vi "do_Weight_Weighing_Machine.vi"(8 "error in (no error)":errorcluster, 11 "Waage_Config":T1={"Enable Termination\nChar (T)"=TRUE, "termination char\n(0xA = '\\n' = LF) "=10, "timeout (10sec)"=3000, "baud rate (9600)"=9600, "data bits (8)"=8, "parity (0:none)"=enum."None", "stop bits (10: 1 bit)"=10, "flow control (0:none)"=0, "Serial Port"=""} {"flow control (0:none)" items=["None", "XON/XOFF", "RTS/CTS", "XON/XOFF & RTS/CTS", "DTR/DSR", "XON/XOFF & DTR/DSR"]; "stop bits (10: 1 bit)" items=["1.0"=10, "1.5"=15, "2.0"=20]}) -> (0 "error out":errorcluster={"status"=TRUE, "code"=-1073807339, "source"="VISA Read in do_Weight_Weighing_Machine.vi"}, 3 "weight(g)":i32)   [LabVIEW 2012]
uses:
  <vilib>/Instr/_visa.llb/VISA Configure Serial Port (Instr).vi
panel:
  out "return count 2":u32=9
  out "return count":u32
  out "read buffer":string
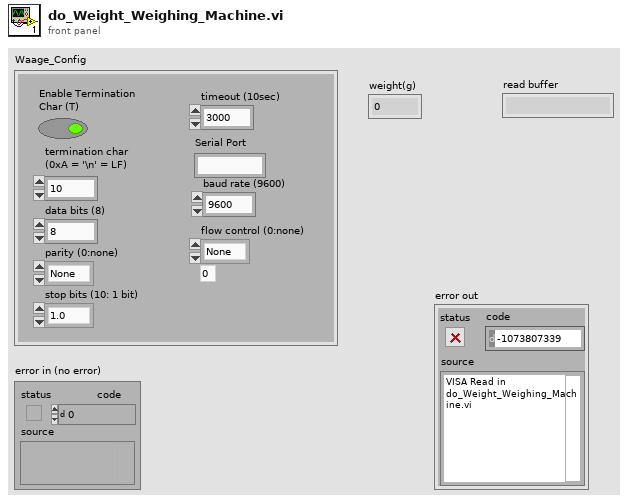
[diagram p1: front panel]
types:
  T1 = cluster{"Enable Termination\nChar (T)":bool, "termination char\n(0xA = '\\n' = LF) ":u8, "timeout (10sec)":u32, "baud rate (9600)":u32, "data bits (8)":u16, "parity (0:none)":enum16{"None", "Odd", "Even", "Mark", "Space"}, "stop bits (10: 1 bit)":u16, "flow control (0:none)":u16, "Serial Port":string}
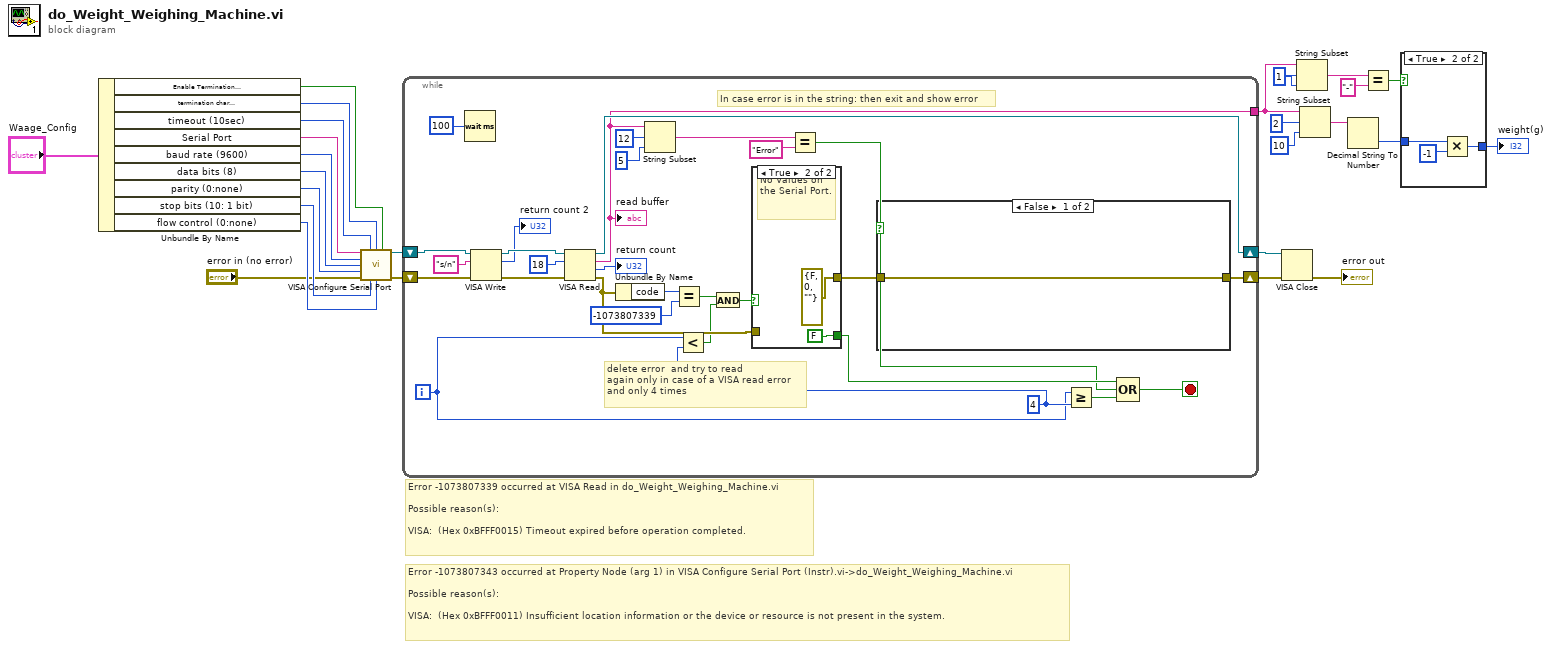
[diagram p0: block diagram]
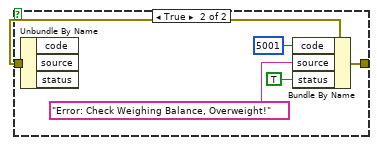
[diagram p3: hidden frame]
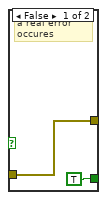
[diagram p4: hidden frame]
diagram:
  w11 = 1 ("offset (0)")
  # "Error -1073807343 occurred at Property Node (arg 1) in VISA Configure Serial Port (Instr).vi->do_Weight_Weighing_Machine.vi\n\nPossible reason(s):\n\nVISA:  (Hex 0xBFFF0011) Insufficient location information or the device or resource is not present in the system."
  # "Error -1073807339 occurred at VISA Read in do_Weight_Weighing_Machine.vi\n\nPossible reason(s):\n\nVISA:  (Hex 0xBFFF0015) Timeout expired before operation completed."
  n1 = Unbundle By Name("Waage_Config") -> ("Enable Termination\nChar (T)"=w22:bool, "termination char\n(0xA = '\\n' = LF)"=w21:u8, "timeout (10sec)"=w20:u32, "Serial Port"=w1:string, "baud rate (9600)"=w19:u32, "data bits (8)"=w18:u16, "parity (0:none)"=w17:enum16{"None", "Odd", "Even", "Mark", "Space"}, "stop bits (10: 1 bit)"=w16:u16, "flow control (0:none)"=w15:u16)
  n2 = call-poly "VISA Configure Serial Port"("VISA resource name"=w1, "timeout (10sec)"=w20, "termination char\n(0xA = '\\n' = LF)"=w21, "Enable Termination\nChar (T)"=w22, "baud rate (9600)"=w19, "data bits (8)"=w18, "parity (0:none)"=w17, "error in (no error)"="error in (no error)", "stop bits (10: 1 bit)"=w16, "flow control (0:none)"=w15) -> ("VISA resource name out"=w26:refnum<visa-resource-name>, "error out"=w25:errorcluster)  [unwired: 4 in]
  n3 = while {
    shift-right: [w47] -> w12
    shift-left: w26 -> [w55]
    shift-right: [w34] -> w24
    shift-left: w25 -> [w54]
    tunnel: [w40] -> w6
    i -> [w29]
    stop <- w41 stop-if-true
    w30 = 4 ("y")
    # "In case error is in the string: then exit and show error"
    # "delete error  and try to read \nagain only in case of a VISA read error\nand only 4 times"
    n4 = Wait (ms)(milliseconds to wait=u32 100) -> ()  [unwired: 1 out]
    n5 = VISA Write(VISA resource name=w55, write buffer="s/n", error in (no error)=w54) -> (VISA resource name out=w53:refnum<visa-resource-name>, return count=→"return count 2":u32, error out=w52:errorcluster)
    n6 = VISA Read(VISA resource name=w53, byte count=u32 18, error in (no error)=w52) -> (VISA resource name out=w47:refnum<visa-resource-name>, read buffer=w40:string, return count=→"return count":u32, error out=w43:errorcluster)
    "read buffer" <- w40
    n7 = Unbundle By Name(w43) -> ("code"=w45:i32)
    n8 = String Subset(string=w40, offset (0)=12, length (rest)=5 ("offset (0)")) -> (substring=w37:string)
    n9 = Equal?(x=w45, y=-1073807339) -> (x = y?=w28:bool)
    n10 = Less?(x=w29, y=w30) -> (x < y?=w31:bool)
    n11 = And(x=w28, y=w31) -> (x .and. y?=w27:bool)
    n12 = case shown="True" w27 {
      tunnel: [TRUE FALSE] -> w42
      tunnel: [w62 errorcluster {"status"=FALSE, "code"=0, "source"=""} ("error IO")] -> w35
      tunnel: w43 -> [w62 _]
      frame False {
        # "a real error occures"
      }
      frame True {
        # "No Values on the Serial Port."
      }
    }
    n13 = Equal?(x=w37, y="Error") -> (x = y?=w33:bool)
    n14 = case shown="False" w33 {
      tunnel: w35 -> [w56 w61]
      tunnel: [w56 w60] -> w34
      frame False {
      }
      frame True {
        n15 = Unbundle By Name(w61) -> ()  [unwired: 3 out]
        n16 = Bundle By Name(cluster=w61, "code"=5001, "source"="Error: Check Weighing Balance, Overweight!", "status"=TRUE) -> (w60:errorcluster)
      }
    }
    n17 = Greater Or Equal?(x=w29, y=w30) -> (x >= y?=w32:bool)
    n18 = Compound Arithmetic op=OR(w42, w33, w32) -> (w41:bool)
  }
  n19 = VISA Close(VISA resource name=w12, error in (no error)=w24) -> (error out=→"error out":errorcluster)
  n20 = String Subset(string=w6, offset (0)=w11, length (rest)=w11) -> (substring=w10:string)
  n21 = String Subset(string=w6, offset (0)=2, length (rest)=10 ("offset (0)")) -> (substring=w4:string)
  n22 = Decimal String To Number(string=w4) -> (number=w3:i32)  [unwired: 2 in, 1 out]
  n23 = Equal?(x=w10, y="-") -> (x = y?=w8:bool)
  n24 = case shown="True" w8 {
    tunnel: w3 -> [w66 w69]
    tunnel: [w66 w67] -> w2
    frame False {
    }
    frame True {
      n25 = Multiply(x=w69, y=-1) -> (x*y=w67:i32)
    }
  }
  "weight(g)" <- w2
